vi "Idle Reference Image Window Management 26_01_18.vi"(6 "Function":T1(ring), 8 "error in (no error)":errorcluster, 11 "UI queue (used with \"Open\")":refnum<queue>) -> (0 "error out":errorcluster)   [LabVIEW 2020]
uses:
  Queue/Message Queue/Typedefs/Message Cluster.ctl
  Global Variables/General Globals.vi
panel:
  out "Time taken":u32
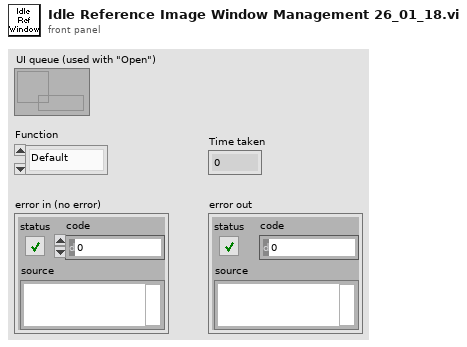
[diagram p1: front panel]
types:
  T1 = enum16{"Default", "Initialize", "Open", "Close", "Exit"}
  T2 = enum32{"Invalid", "Standard", "Closed", "Hidden", "Minimized", "Maximized"}
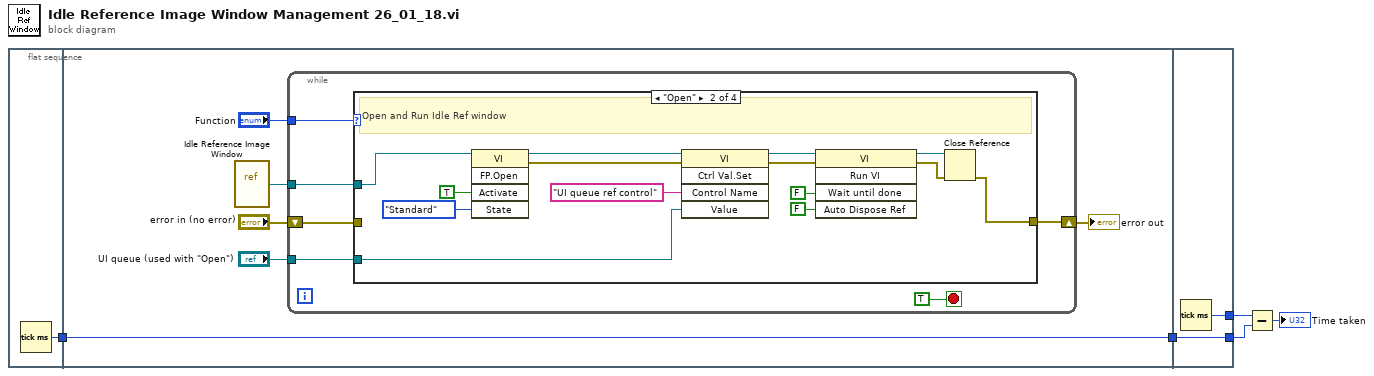
[diagram p0: block diagram]
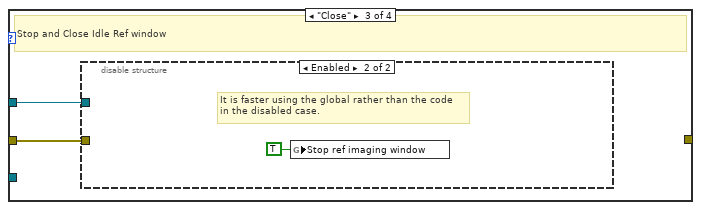
[diagram p3: hidden frame]
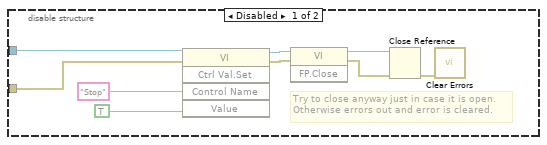
[diagram p4: hidden frame]
diagram:
  n1 = flat-sequence {
    tunnel: [w6] -> w4
    tunnel: w4 -> [w7]
    tunnel: [w7] -> w3
    tunnel: [w47] -> w5
    tunnel: w3 -> [w46]
    tunnel: [w46] -> w2
    frame #0 {
      n2 = Tick Count (ms)() -> (millisecond timer value=w6:u32)
    }
    frame #1 {
      n3 = vi-ref "Idle Reference Image Window.vi"() -> (w10:refnum<vi>)
      n4 = while {
        tunnel: "Function" -> [w18]
        shift-right: [w16] -> w9
        shift-left: "error in (no error)" -> [w15]
        tunnel: w10 -> [w14]
        tunnel: "UI queue (used with \"Open\")" -> [w13]
        stop <- TRUE stop-if-true
        n5 = case shown="\"Open\"" w18 {
          tunnel: w15 -> [w19 _ w35 _]
          tunnel: [w19 w20 _ _] -> w16
          tunnel: w14 -> [_ w29 w34 _]
          tunnel: w13 -> [_ w22 _ _]
          frame Default {
          }
          frame "Open" {
            # "Open and Run Idle Ref window"
            n6 = invoke class="VI" method="FP.Open"(reference=w29, "Activate"=TRUE ("Activate?"), "State"=T2."Standard") -> (reference out=w26:refnum<vi>, error out=w24:errorcluster)  [unwired: 2 in, 3 out]
            n7 = invoke class="VI" method="Ctrl Val.Set"(reference=w26, error in=w24, "Control Name"="UI queue ref control", "Value"=w22) -> (reference out=w25:refnum<vi>, error out=w23:errorcluster)  [unwired: 1 in, 3 out]
            n8 = invoke class="VI" method="Run VI"(reference=w25, error in=w23, "Wait until done"=FALSE ("Wait Until Done"), "Auto Dispose Ref"=FALSE ("Auto Dispose Reference")) -> (reference out=w28:refnum<vi>, error out=w27:errorcluster)  [unwired: 1 in, 3 out]
            n9 = Close Reference(reference=w28, error in (no error)=w27) -> (error out=w20:errorcluster)
          }
          frame "Close" {
            # "Stop and Close Idle Ref window"
            n10 = disable-structure shown="Enabled" {
              disable-tunnel: w35 -> [w44 _]
              disable-tunnel: w34 -> [w41 _]
              frame Disabled {
                # "Try to close anyway just in case it is open.\nOtherwise errors out and error is cleared."
                n11 = invoke class="VI" method="Ctrl Val.Set"(reference=w41, error in=w44, "Control Name"="Stop", "Value"=TRUE) -> (reference out=w36:refnum<vi>, error out=w37:errorcluster)  [unwired: 1 in, 3 out]
                n12 = invoke class="VI" method="FP.Close"(reference=w36, error in=w37) -> (reference out=w40:refnum<vi>, error out=w39:errorcluster)  [unwired: 1 in, 1 out]
                n13 = Close Reference(reference=w40, error in (no error)=w39) -> (error out=w38:errorcluster)
                n14 = call <vilib>:"Clear Errors.vi"("error in (no error)"=w38) -> ()  [unwired: 5 in, 2 out]
              }
              frame Enabled {
                # "It is faster using the global rather than the code\nin the disabled case."
                n15 = global write "General Globals.vi" "Stop ref imaging window"(TRUE ("Stop ref imaging window")) -> ()
              }
            }
          }
          frame "Exit" {
          }
        }
      }
      "error out" <- w9
    }
    frame #2 {
      n16 = Tick Count (ms)() -> (millisecond timer value=w47:u32)
    }
  }
  n17 = Subtract(x=w5, y=w2) -> (x-y=→"Time taken":u32)
